vi "subturnOnLedForNSec.vi"(8 "Second":dbl, 9 "Pin Number":dbl, 11 "Arduino Resource":T1={"VISA resource"="", "Board Type"=enum."Uno", "Connection Type"=enum."USB / Serial", "Bytes Per Packet (15)"=15}) -> (3 "Arduino Resource 2":T1={"VISA resource"="", "Board Type"=enum."Uno", "Connection Type"=enum."USB / Serial", "Bytes Per Packet (15)"=15})   [LabVIEW 2016]
uses:
  <vilib>/LabVIEW Interface for Arduino/Type Defs/Arduino Resource.ctl
  <vilib>/LabVIEW Interface for Arduino/Type Defs/Board Type.ctl
  <vilib>/LabVIEW Interface for Arduino/LabVIEW Interface for Arduino.lvlib
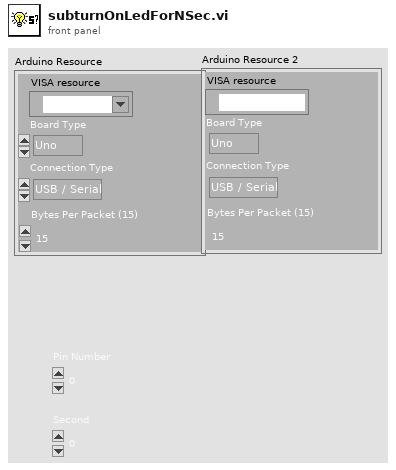
[diagram p1: front panel]
types:
  T1 = typedef "LabVIEW Interface for Arduino.lvlib/Arduino Resource.ctl" = cluster{"VISA resource":refnum<visa-resource-name>, "Board Type":T2, "Connection Type":enum8{"USB / Serial"}, "Bytes Per Packet (15)":u8}
  T2 = typedef "LabVIEW Interface for Arduino.lvlib/Board Type.ctl" = enum16{"Uno", "Dimuelanove w/Atmega 328", "Mega 2560"}
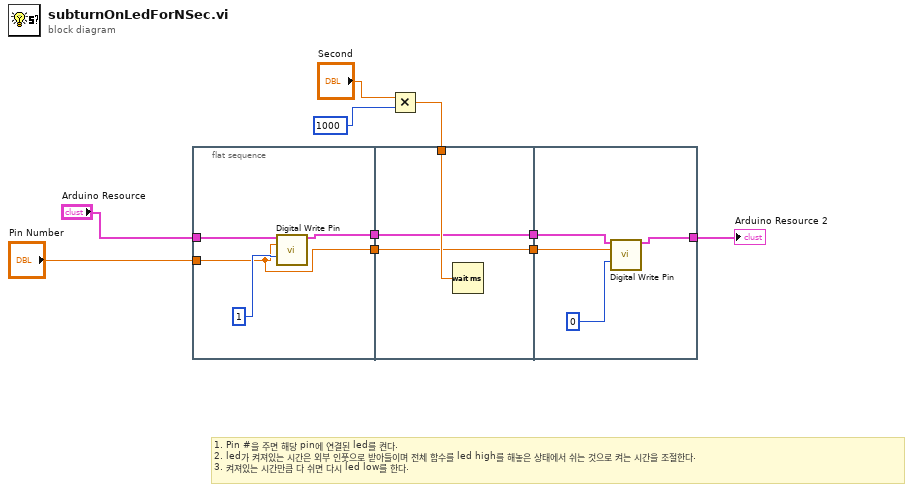
[diagram p0: block diagram]
diagram:
  # "1. Pin #을 주면 해당 pin에 연결된 led를 켠다. \n2. led가 켜져있는 시간은 외부 인풋으로 받아들이며 전체 함수를 led high를 해놓은 상태에서 쉬는 것으로 켜는 시간을 조절한다.\n3. 켜져있는 시간만큼 다 쉬면 다시 led low를 한다."
  n1 = flat-sequence {
    tunnel: "Arduino Resource" -> [w14]
    tunnel: "Pin Number" -> [w11]
    tunnel: [w12] -> w4
    tunnel: [w11] -> w2
    tunnel: w8 -> [w17]
    tunnel: [w16] -> w5
    tunnel: w4 -> [w16]
    tunnel: [w15] -> w3
    tunnel: w2 -> [w15]
    tunnel: w5 -> [w21]
    tunnel: w3 -> [w19]
    tunnel: [w18] -> w1
    frame #0 {
      n2 = call <vilib>:"Digital Write Pin.vi"("Arduino Resource"=w14, "Digital I/O Pin (0)"=w11, "Value (0)"=1) -> ("Arduino Resource"=w12:T1)  [unwired: 11 in, 1 out]
    }
    frame #1 {
      n3 = Wait (ms)(milliseconds to wait=w17) -> ()  [unwired: 1 out]
    }
    frame #2 {
      n4 = call <vilib>:"Digital Write Pin.vi"("Arduino Resource"=w21, "Digital I/O Pin (0)"=w19, "Value (0)"=0) -> ("Arduino Resource"=w18:T1)  [unwired: 11 in, 1 out]
    }
  }
  n5 = Multiply(x="Second", y=1000) -> (x*y=w8:dbl)
  "Arduino Resource 2" <- w1
